vi "Read Attribute (String).vi"(8 "error in":errorcluster, 10 "Attribute Name":string, 11 "node in":refnum<k20>) -> (0 "error out":errorcluster, 1 "value":string, 3 "node out":refnum<k20>)   [LabVIEW 2020, in "AIM ARINC 664 Import.lvlib"]
uses:
  AIM ARINC 664 Import.lvlib
  <resource>/objmgr/DOMUserDefRef.rc
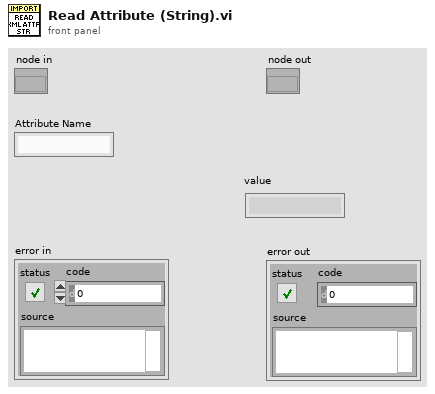
[diagram p1: front panel]
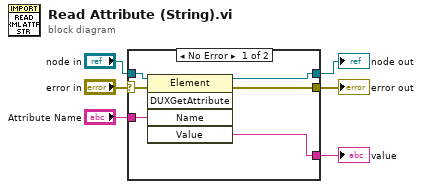
[diagram p0: block diagram]
diagram:
  n1 = case shown="No Error" "error in" {
    selector: "error in" -> [w8 w14]
    tunnel: [w9 w14] -> w6
    tunnel: "node in" -> [w11 w13]
    tunnel: "Attribute Name" -> [w12 _]
    tunnel: [w7 _] -> w1
    tunnel: [w10 w13] -> w3
    frame No Error {
      n2 = invoke class="Element" method="DUXGetAttribute"(reference=w11, error in=w8, "Name"=w12) -> (reference out=w10:refnum<k20>, error out=w9:errorcluster, "Value"=w7:string)  [unwired: 2 in, 2 out]
    }
    frame Error {
    }
  }
  "error out" <- w6
  "node out" <- w3
  "value" <- w1
